vi "Status.Simple Text Status Indicator.vi"(7 "Show OK Indication":bool, 8 "error in":errorcluster, 11 "Status TextBox":refnum<vi>) -> (0 "error out":errorcluster)   [LabVIEW 2024, in "EQMF.lvlib" / "Status Utils.lvlib"]
uses:
  Status Utils.lvlib
panel:
  in  "Test":bool
  out "InsX Status":string caption="InstrumentX"
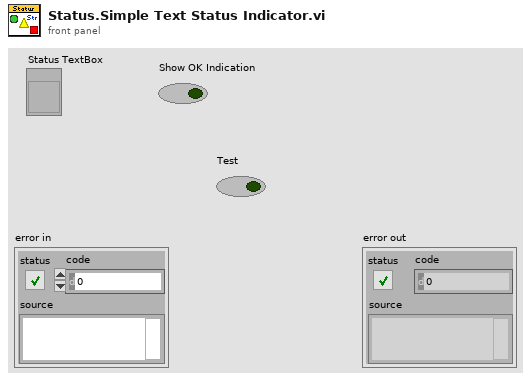
[diagram p1: front panel]
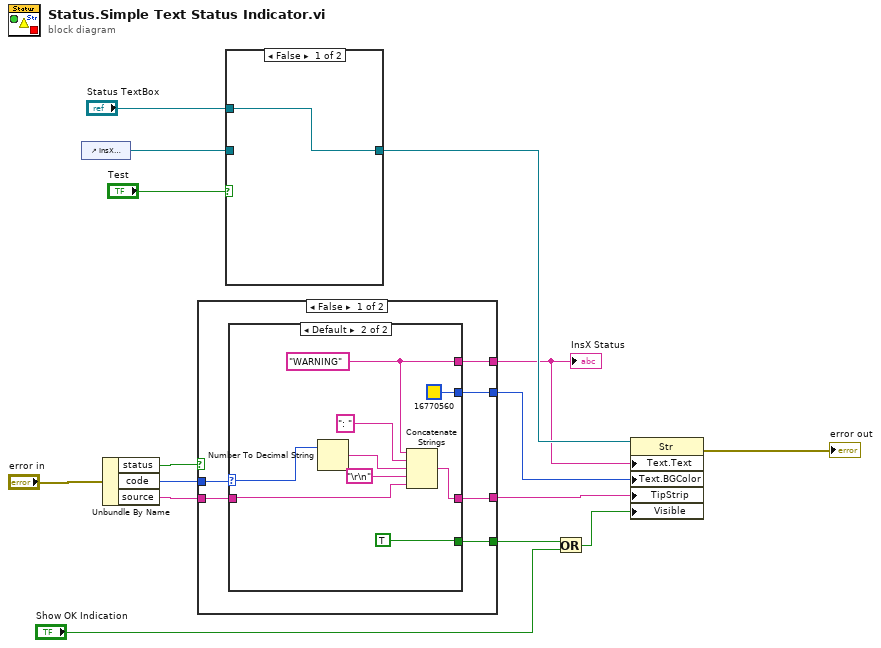
[diagram p0: block diagram]
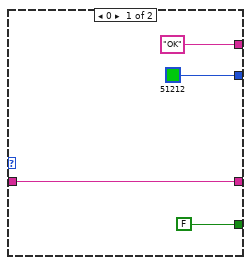
[diagram p2: hidden frame]
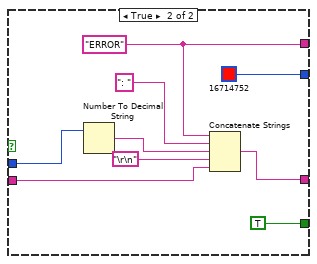
[diagram p3: hidden frame]
diagram:
  n1 = control-ref of="InsX Status"() -> (w14:refnum<vi>)
  n2 = Unbundle By Name("error in") -> ("status"=w12:bool, "code"=w11:i32, "source"=w9:string)
  n3 = case shown="False" w12 {
    tunnel: w11 -> [w21 w42]
    tunnel: [w20 u32 16714752] -> w10
    tunnel: w9 -> [w19 w39]
    tunnel: [w18 w38] -> w8
    tunnel: [w17 w37] -> w4
    tunnel: [w16 TRUE] -> w2
    frame False {
      n4 = case shown="Default" w21 {
        selector: w21 -> [_ w31]
        tunnel: [u32 51212 u32 16770560] -> w20
        tunnel: w19 -> [w24 w30]
        tunnel: [w24 w29] -> w18
        tunnel: ["OK" w27] -> w17
        tunnel: [FALSE TRUE] -> w16
        frame 0 {
        }
        frame Default {
          w27 = "WARNING"
          n5 = Number To Decimal String(number=w31) -> (decimal integer string=w33:string)  [unwired: 1 in]
          n6 = Concatenate Strings(w27, ": ", w33, "\r\n", w30) -> (w29:string)
        }
      }
    }
    frame True {
      w37 = "ERROR"
      n7 = Number To Decimal String(number=w42) -> (decimal integer string=w41:string)  [unwired: 1 in]
      n8 = Concatenate Strings(w37, ": ", w41, "\r\n", w39) -> (w38:string)
    }
  }
  "InsX Status" <- w4
  n9 = case shown="False" "Test" {
    tunnel: "Status TextBox" -> [w44 _]
    tunnel: w14 -> [_ w45]
    tunnel: [w44 w45] -> w5
    frame False {
    }
    frame True {
    }
  }
  n10 = Or(x=w2, y="Show OK Indication") -> (x .or. y?=w3:bool)
  n11 = property on="Property Node" class="Str"(reference=w5, "Text.Text"=w4, "Text.BGColor"=w10, "TipStrip"=w8, "Visible"=w3) -> (error out=→"error out":errorcluster)  [unwired: 1 in, 1 out]
